vi "3_Configuration.vi"(0 "Disabled":T1(ring)) -> ()   [LabVIEW 2015]
panel:
  in  "Increment":dbl
  in  "Increment Rate":dbl
  in  "Target RPM":dbl
  in  "Test Type":u16(ring) items=["Sweep", "Step"]
  in  "Report File Path":path
  in  "Test ID":string
  in  "Torque Tolerance ±":dbl
  in  "Nominal Torque (N-m)":dbl
  in  "Temp Tolerance ±":dbl
  in  "Speed Tolerance ±":dbl
  in  "Flow Tolerance ±":dbl
  in  "Pump SN":string
  in  "Nominal Temp (deg C)":dbl
  in  "Nominal Flow (LPM)":dbl
  in  "Nominal Speed (RPM)":dbl
  in  "Model":string
  in  "Copy":bool
  in  "Test Window":bool
  in  "Cancel":bool
  in  "Save":bool
  # "Developed by: VR Engineers"
  # "Contact: 9891971134"
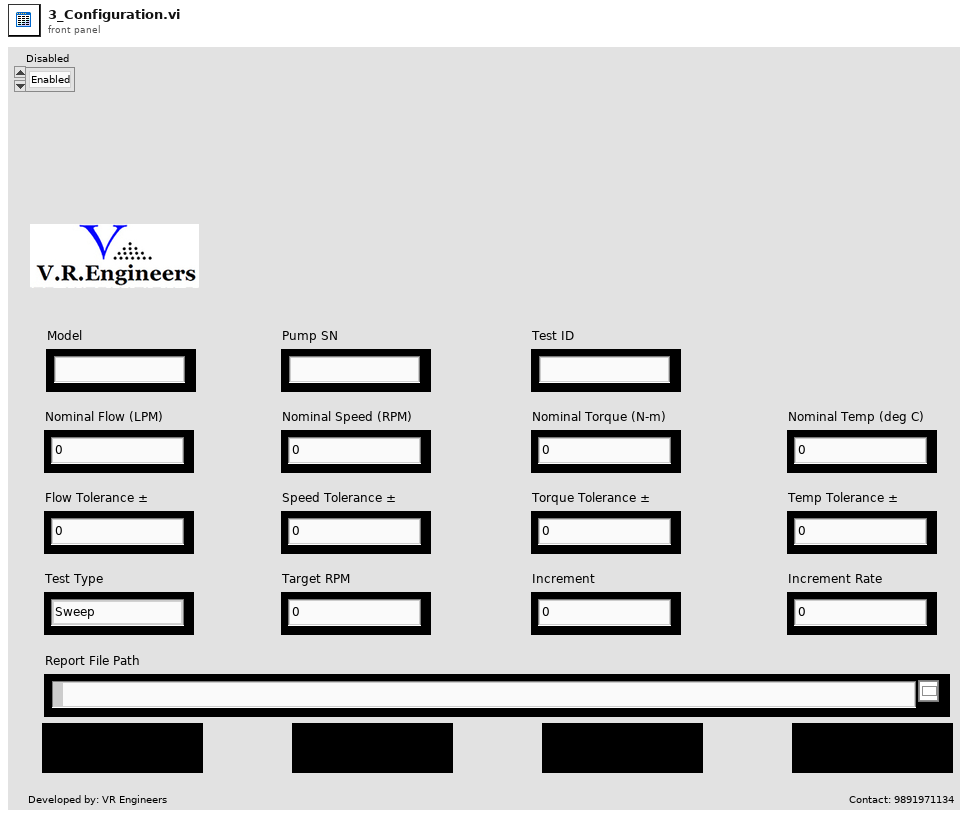
[diagram p1: front panel]
types:
  T1 = enum8{"Enabled", "Disabled", "Disabled and Grayed Out"}
  T2 = cluster{"Model":string, "Pump SN":string, "Test ID":string, "Nominal Speed (RPM)":dbl, "Nominal Flow (LPM)":dbl, "Nominal Temp (deg C)":dbl, "Speed Tolerance (%)":dbl, "Flow Tolerance (%)":dbl, "Temp Tolerance(%)":dbl, "Nominal Torque (N-m)":dbl, "Torque Tolerance (%)":dbl, "Report File Path":path, "Test Type":u16, "Target RPM":dbl, "Increment":dbl, "Increment Rate":dbl}
  T3 = enum16{"open", "replace", "create", "open or create", "replace or create", "replace or create with confirmation"}
  T4 = enum16{"big-endian, network order", "native, host order", "little-endian"}
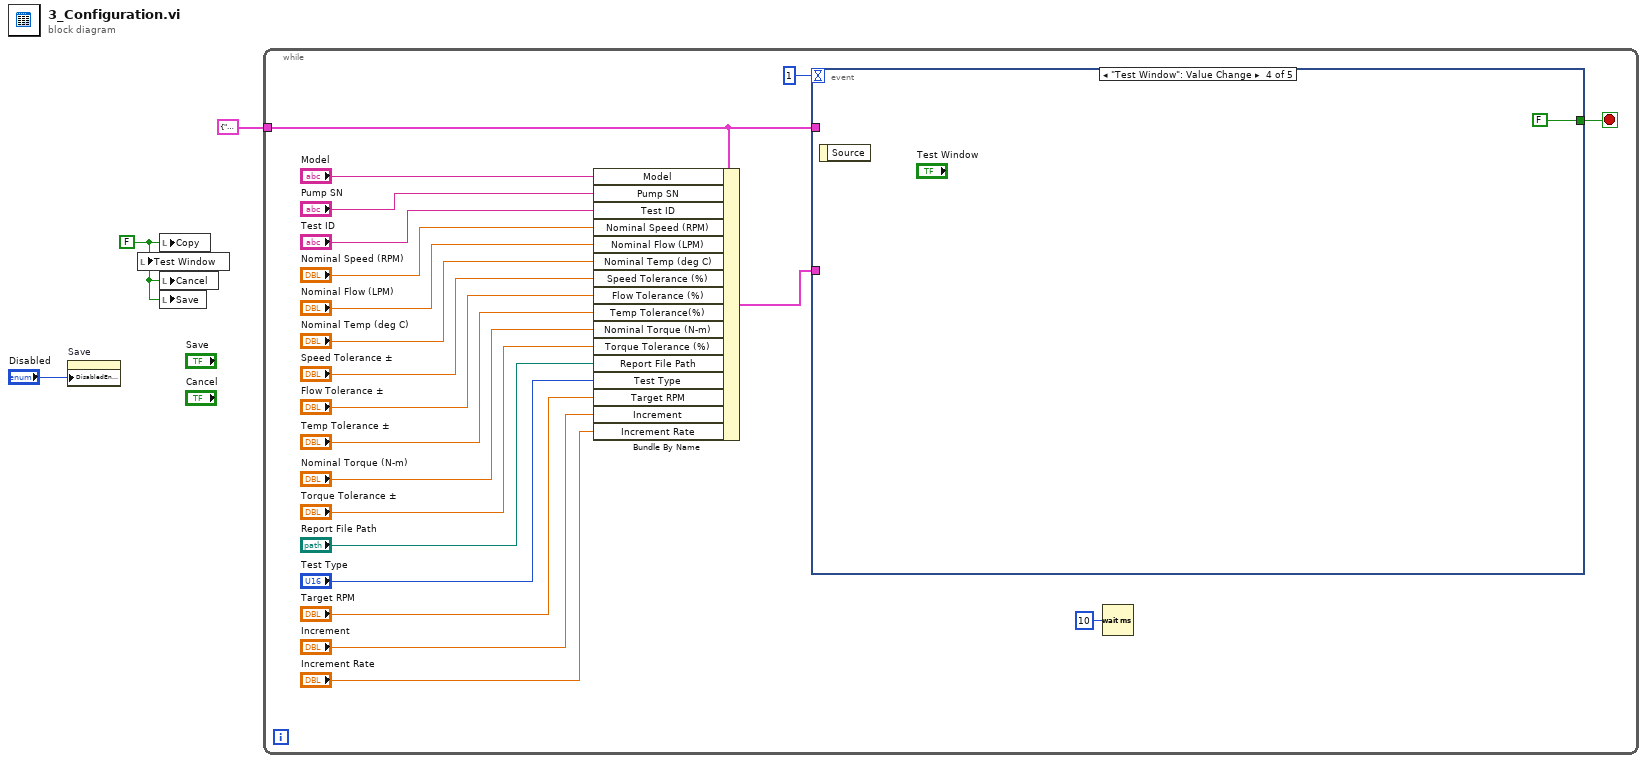
[diagram p0: block diagram]
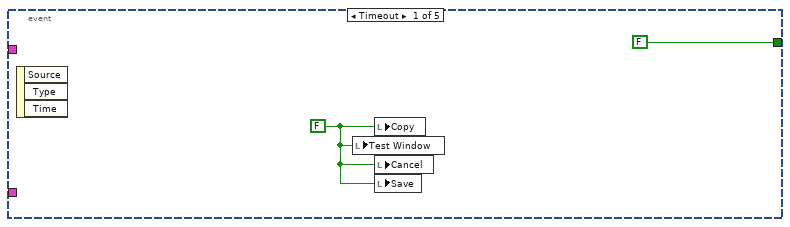
[diagram p2: hidden frame]
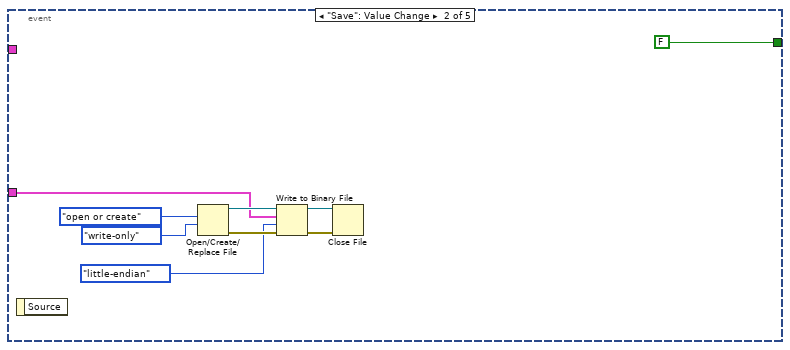
[diagram p3: hidden frame]
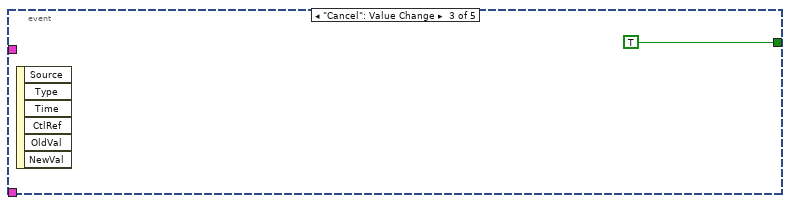
[diagram p4: hidden frame]
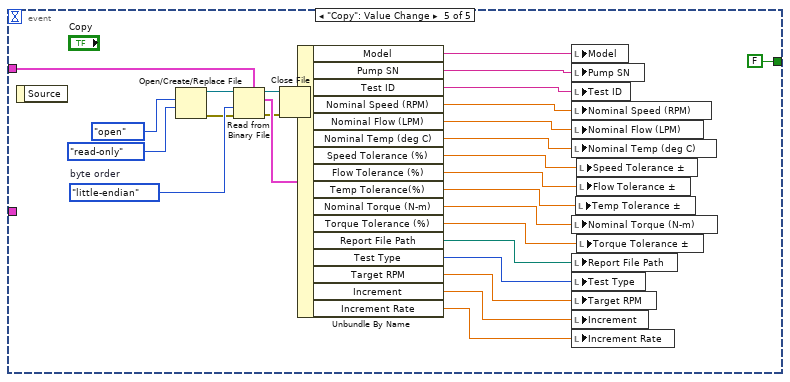
[diagram p5: hidden frame]
diagram:
  w3 = FALSE ("Copy")
  n1 = property on="Save" class="Bool (strict)"("DisabledEnum"="Disabled") -> ()  [unwired: 2 in, 2 out]
  n2 = local write "Test Window"(w3) -> ()
  n3 = local write "Copy"(w3) -> ()
  n4 = local write "Cancel"(w3) -> ()
  n5 = local write "Save"(w3) -> ()
  n6 = while {
    tunnel: T2 {"Model"="", "Pump SN"="", "Test ID"="", "Nominal Speed (RPM)"=0.0, "Nominal Flow (LPM)"=0.0, "Nominal Temp (deg C)"=0.0, "Speed Tolerance (%)"=0.0, "Flow Tolerance (%)"=0.0, "Temp Tolerance(%)"=0.0, "Nominal Torque (N-m)"=0.0, "Torque Tolerance (%)"=0.0, "Report File Path"=path "", "Test Type"=0, "Target RPM"=0.0, "Increment"=0.0, "Increment Rate"=0.0} -> [w9]
    stop <- w22 stop-if-true
    n7 = Bundle By Name(cluster=w9, "Model"="Model", "Pump SN"="Pump SN", "Test ID"="Test ID", "Nominal Speed (RPM)"="Nominal Speed (RPM)", "Nominal Flow (LPM)"="Nominal Flow (LPM)", "Nominal Temp (deg C)"="Nominal Temp (deg C)", "Speed Tolerance (%)"="Speed Tolerance ±", "Flow Tolerance (%)"="Flow Tolerance ±", "Temp Tolerance(%)"="Temp Tolerance ±", "Nominal Torque (N-m)"="Nominal Torque (N-m)", "Torque Tolerance (%)"="Torque Tolerance ±", "Report File Path"="Report File Path", "Test Type"="Test Type", "Target RPM"="Target RPM", "Increment"="Increment", "Increment Rate"="Increment Rate") -> (w21:T2)
    n8 = event shown="[3] \"Test Window\": Value Change" {
      selector: _ -> [_ _ _ _ _]
      dyn-events: _ -> [_ _ _ _ _]
      timeout: 1 -> [_ _ _ _ _]
      tunnel: [FALSE ("status") FALSE ("status") TRUE ("status") FALSE ("status") FALSE ("status")] -> w22
      tunnel: w21 -> [_ w27 _ _ _]
      tunnel: w9 -> [_ _ _ _ w57]
      event Timeout {
        w25 = FALSE ("Copy")
        n9 = event-data() -> ()  [unwired: 1 in, 3 out]
        n10 = local write "Test Window"(w25) -> ()
        n11 = local write "Copy"(w25) -> ()
        n12 = local write "Cancel"(w25) -> ()
        n13 = local write "Save"(w25) -> ()
      }
      event "Save": Value Change {
        n14 = event-data() -> ()  [unwired: 1 in, 1 out]
        n15 = Open/Create/Replace File(operation (0:open)=T3."open or create", access (0:read/write)=enum16{"read/write", "read-only", "write-only"}."write-only") -> (refnum out=w34:refnum<file>, error out=w35:errorcluster)  [unwired: 4 in, 1 out]
        n16 = Write to Binary File(file (use dialog)=w34, data=w27, error in=w35, 9:T4."little-endian" ("byte order")) -> (refnum out=w29:refnum<file>, error out=w30:errorcluster)  [unwired: 2 in, 1 out]
        n17 = Close File(refnum=w29, error in=w30) -> ()  [unwired: 2 out]
      }
      event "Cancel": Value Change {
        n18 = event-data() -> ()  [unwired: 1 in, 6 out]
      }
      event "Test Window": Value Change {
        n19 = event-data() -> ()  [unwired: 1 in, 1 out]
      }
      event "Copy": Value Change {
        w61 = T4."little-endian"  # byte order
        n20 = event-data() -> ()  [unwired: 1 in, 1 out]
        n21 = Open/Create/Replace File(operation (0:open)=T3."open", access (0:read/write)=enum16{"read/write", "read-only", "write-only"}."read-only") -> (refnum out=w58:refnum<file>, error out=w59:errorcluster)  [unwired: 4 in, 1 out]
        n22 = Read from Binary File(5:w57, 8:w59, 9:w61, 11:w58) -> (0:w38:errorcluster, 2:w56:T2, 3:w39:refnum<file>)  [unwired: 2 in, 1 out]
        n23 = Close File(refnum=w39, error in=w38) -> ()  [unwired: 2 out]
        n24 = Unbundle By Name(w56) -> ("Model"=w55:string, "Pump SN"=w54:string, "Test ID"=w53:string, "Nominal Speed (RPM)"=w52:dbl, "Nominal Flow (LPM)"=w51:dbl, "Nominal Temp (deg C)"=w50:dbl, "Speed Tolerance (%)"=w49:dbl, "Flow Tolerance (%)"=w48:dbl, "Temp Tolerance(%)"=w47:dbl, "Nominal Torque (N-m)"=w46:dbl, "Torque Tolerance (%)"=w45:dbl, "Report File Path"=w44:path, "Test Type"=w43:u16, "Target RPM"=w42:dbl, "Increment"=w41:dbl, "Increment Rate"=w40:dbl)
        n25 = local write "Model"(w55) -> ()
        n26 = local write "Pump SN"(w54) -> ()
        n27 = local write "Test ID"(w53) -> ()
        n28 = local write "Nominal Speed (RPM)"(w52) -> ()
        n29 = local write "Nominal Flow (LPM)"(w51) -> ()
        n30 = local write "Nominal Temp (deg C)"(w50) -> ()
        n31 = local write "Nominal Torque (N-m)"(w46) -> ()
        n32 = local write "Report File Path"(w44) -> ()
        n33 = local write "Test Type"(w43) -> ()
        n34 = local write "Target RPM"(w42) -> ()
        n35 = local write "Increment"(w41) -> ()
        n36 = local write "Increment Rate"(w40) -> ()
        n37 = local write "Temp Tolerance ±"(w47) -> ()
        n38 = local write "Speed Tolerance ±"(w49) -> ()
        n39 = local write "Flow Tolerance ±"(w48) -> ()
        n40 = local write "Torque Tolerance ±"(w45) -> ()
      }
    }
    n41 = Wait (ms)(milliseconds to wait=u32 10) -> ()  [unwired: 1 out]
  }
